vi "CRYPEAQ GroupCB.vi"(8 "Version":u16(ring) items=["Basic", "Advance", "My"], 9 "NF":dbl=2048.0, 10 "X2":dbl[](array[numeric]), 11 "Fs":dbl=48000.0) -> (0 "Nc":i32, 2 "fc":dbl[](array[numeric]), 3 "Eb":dbl[](array[numeric]))   [LabVIEW 2013]
panel:
  out "Waveform Graph 2":dbl[](graph)
  out "Waveform Graph":dbl[](graph)
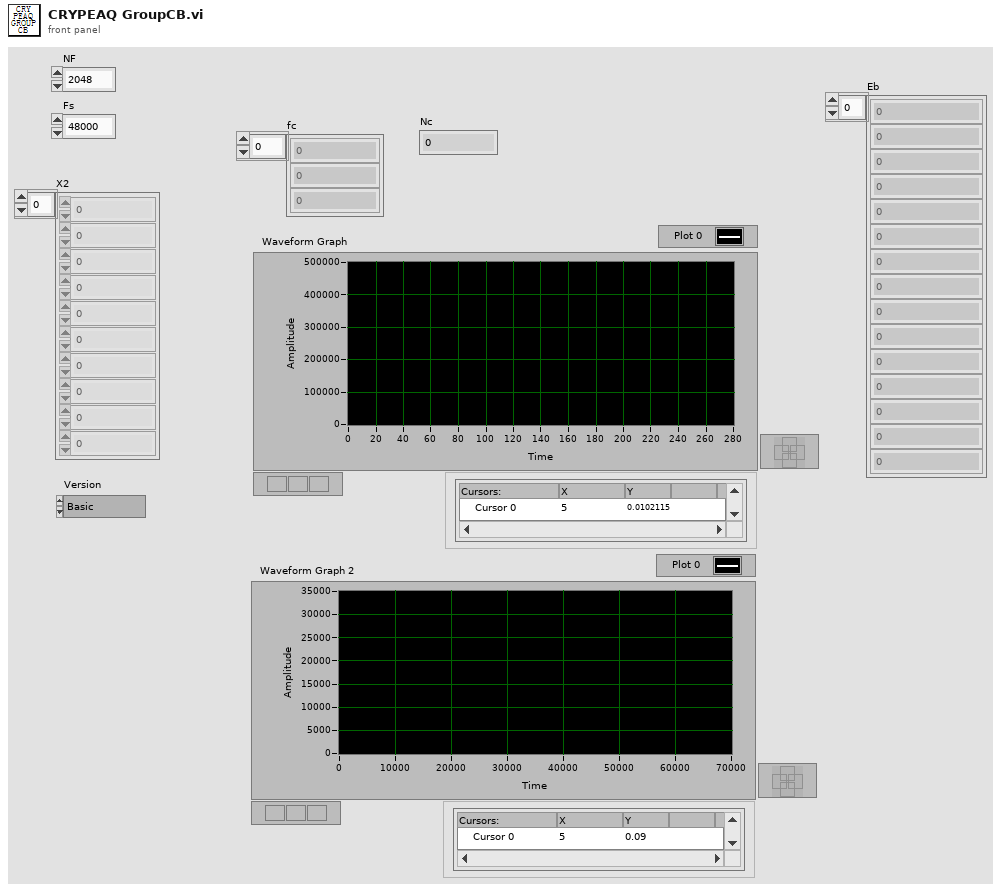
[diagram p1: front panel]
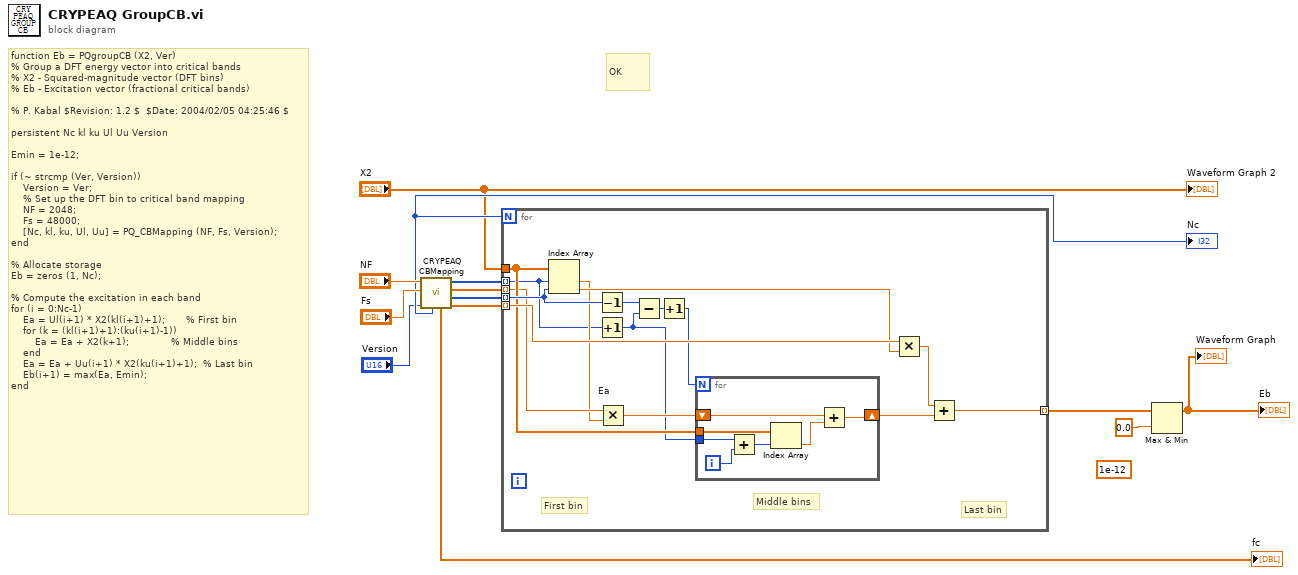
[diagram p0: block diagram]
diagram:
  (unwired) 1e-12 ("x+y")
  # "OK"
  # "function Eb = PQgroupCB (X2, Ver)\n% Group a DFT energy vector into critical bands\n% X2 - Squared-magnitude vector (DFT bins)\n% Eb - Excitation vector (fractional critical bands)\n\n% P. Kabal $Revision: 1.2 $  $Date: 2004/02/05 04:25:46 $\n\npersistent Nc kl ku Ul Uu Version\n\nEmin = 1e-12;\n\nif (~ strcmp (Ver, Version))\n    Version = Ver;\n    % Set up the DFT bin to critical band mapping\n    NF = 2048;\n    Fs = 48000;\n    [Nc, kl, ku, Ul, Uu] = PQ_CBMapping (NF, Fs, Version);\nend\n\n% Allocate storage\nEb = zeros (1, Nc);\n\n% Compute the excitation in each band\nfor (i = 0:Nc-1)\n    Ea = Ul(i+1) * X2(kl(i+1)+1);       % First bin\n    for (k = (kl(i+1)+1):(ku(i+1)-1))\n        Ea = Ea + X2(k+1);              % Middle bins\n    end\n    Ea = Ea + Uu(i+1) * X2(ku(i+1)+1);  % Last bin\n    Eb(i+1) = max(Ea, Emin);\nend"
  n1 = call "CRYPEAQ CBMapping.vi"("Version"="Version", "Fs"="Fs", "NF"="NF") -> ("Uu"=w3:dbl[], "ku"=w5:i32[], "Ul"=w8:dbl[], "kl"=w6:i32[], "fc"=→"fc":dbl[], "Nc"=w9:i32)  [unwired: 1 in, 2 out]
  "Nc" <- w9
  n2 = for {
    N: w9 -> [_]
    tunnel: "X2" -> [w25]
    tunnel: w8 -> [w20] mode=indexing
    tunnel: w6 -> [w18] mode=indexing
    tunnel: w5 -> [w28] mode=indexing
    tunnel: w3 -> [w26] mode=indexing
    tunnel: [w23] -> w13 mode=indexing
    # "Last bin"
    # "Middle bins"
    # "First bin"
    n3 = Index Array(array=w25, index #1=w18, index #2=w28) -> (element #1=w19:dbl, element #2=w24:dbl)
    n4 = Decrement(x=w28) -> (x-1=w27:i32)
    n5 = Increment(x=w18) -> (x+1=w16:i32)
    n6 = Multiply "Ea"(x=w20, y=w19) -> (x*y=w17:dbl)
    n7 = Subtract(x=w27, y=w16) -> (x-y=w15:i32)
    n8 = Increment(x=w15) -> (x+1=w14:i32)
    n9 = for {
      N: w14 -> [_]
      shift-right: [w34] -> w21
      shift-left: w17 -> [w35]
      tunnel: w16 -> [w30]
      tunnel: w25 -> [w33]
      i -> [w31]
      n10 = Add(x=w30, y=w31) -> (x+y=w29:i32)
      n11 = Index Array(array=w33, index=w29) -> (element=w32:dbl)
      n12 = Add(x=w35, y=w32) -> (x+y=w34:dbl)
    }
    n13 = Multiply(x=w26, y=w24) -> (x*y=w22:dbl)
    n14 = Add(x=w22, y=w21) -> (x+y=w23:dbl)
  }
  n15 = Max & Min(x=w13, y=0.0 ("x+y")) -> (max(x,y)=→"Eb" →"Waveform Graph":dbl[])  [unwired: 1 out]
  "Waveform Graph 2" <- "X2"
